vi "Handling Return Tuples.vi"() -> ()   [LabVIEW 2020, in "OPI.lvclass"]
uses:
  OPI.lvclass
  Typedefs/Cmd Line Mode.ctl
  Get Return/Get Return - Pythonic.vi
  From Pythonic/From Pythonic - Tuple.vi
  From Pythonic/From Pythonic - Float.vi
  From Pythonic/From Pythonic - Integer.vi
  From Pythonic/From Pythonic - Boolean.vi
  From Pythonic/From Pythonic - String.vi
panel:
  out "Float":dbl
  out "Integer":i64
  out "Return Value":bool caption="Boolean"
  out "String":string
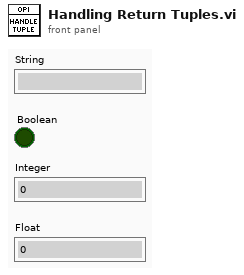
[diagram p1: front panel]
types:
  T1 = typedef "OPI.lvclass/Cmd Line Mode.ctl" = enum16{"Debug", "Hidden"}
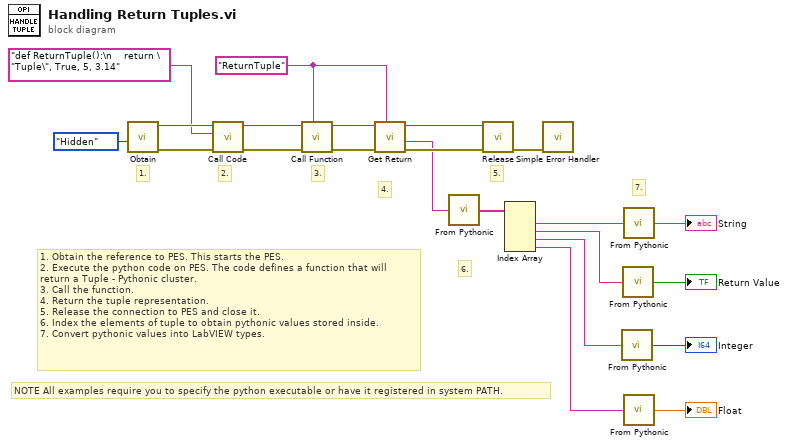
[diagram p0: block diagram]
diagram:
  w13 = "ReturnTuple" ("Function")
  # "NOTE All examples require you to specify the python executable or have it registered in system PATH."
  # "1. Obtain the reference to PES. This starts the PES.\n2. Execute the python code on PES. The code defines a function that will\nreturn a Tuple - Pythonic cluster.\n3. Call the function.\n4. Return the tuple representation.\n5. Release the connection to PES and close it.\n6. Index the elements of tuple to obtain pythonic values stored inside.\n7. Convert pythonic values into LabVIEW types."
  # "7."
  # "6."
  # "5."
  # "4."
  # "3."
  # "2."
  # "1."
  n1 = call "Obtain.vi"("Cmd Line Mode (Hidden)"=Cmd_Line_Mode."Hidden") -> ("Error Out"=w21:errorcluster, "OPI Ref"=w22:refnum<data-value>)  [unwired: 9 in]
  n2 = call "Call Code.vi"("Error In"=w21, "Pythonic Code"="def ReturnTuple():\n    return \"Tuple\", True, 5, 3.14", "OPI Ref"=w22) -> ("Error Out"=w18:errorcluster, "OPI Ref"=w19:refnum<data-value>)  [unwired: 7 in]
  n3 = call "Call Function.vi"("Function Name"=w13, "Error In"=w18, "OPI Ref"=w19) -> ("Error Out"=w14:errorcluster, "OPI Ref"=w15:refnum<data-value>)  [unwired: 7 in]
  n4 = call-poly "Get Return.vi"("Function Name"=w13, "Error In"=w14, "OPI Ref"=w15) -> ("Error Out"=w8:errorcluster, "Pythonic Return Value"=w6:string, "OPI Ref"=w17:refnum<data-value>)  [unwired: 6 in]
  n5 = call-poly "From Pythonic.vi"("Pythonic Value"=w6) -> ("Tuple"=w1:string[])  [unwired: 4 in]
  n6 = call "Release.vi"("Error In"=w8, "OPI Ref"=w17) -> ("Error Out"=w7:errorcluster)  [unwired: 9 in]
  n7 = Index Array(array=w1) -> (element #1=w5:string, element #2=w4:string, element #3=w3:string, element #4=w2:string)  [unwired: 4 in]
  n8 = call <vilib>:"Simple Error Handler.vi"("error in (no error)"=w7) -> ()  [unwired: 4 in, 5 out]
  n9 = call-poly "From Pythonic.vi"("Pythonic Value"=w3) -> ("Integer"=→"Integer":i64)  [unwired: 4 in]
  n10 = call-poly "From Pythonic.vi"("Pythonic Value"=w4) -> ("Boolean"=→"Return Value":bool)  [unwired: 4 in]
  n11 = call-poly "From Pythonic.vi"("Pythonic Value"=w5) -> ("String"=→"String":string)  [unwired: 4 in]
  n12 = call-poly "From Pythonic.vi"("Pythonic Value"=w2) -> ("Float"=→"Float":dbl)  [unwired: 4 in]
